vi "Handle Last Ack Core.vi"(4 "error in (no error)":errorcluster, 6 "Last Ack":refnum<class "Last Ack.lvclass">, 7 "TestStand Controller in":refnum<class "Controller API.lvclass">) -> (0 "error out":errorcluster, 3 "TestStand Controller out":refnum<class "Controller API.lvclass">)   [LabVIEW 2016, in "Controller API.lvlib" / "Controller API.lvclass"]
doc: "(<B>Filename</B>: Actor Framework.lvlib:Actor.lvclass:Handle Last Ack Core.vi)\n\nDefines how the caller actor responds to the Last Ack message from a nested actor. The Last Ack message is the final message a nested actor sends to its caller before it shuts down. The message contains information about the final state of the nested actor.\n\nBy default, this method does nothing except return any error the nested actor sent. A descendant class may override this method to define behavior."
uses:
  <userlib>/Measurement Utility API/Controller API.lvclass
  <vilib>/ActorFramework/LastAck/Last Ack.lvclass
  <userlib>/Common Components/Measurement Actor/Measurement.lvclass
  <vilib>/ActorFramework/LastAck/Last Ack.lvclass/Last Ack.ctl
  <userlib>/Common Components/Results/Results.lvclass
  <userlib>/Common Components/Measurement Actor/Measurement.lvclass/Measurement.ctl
  <userlib>/Measurement Utility API/Controller API.lvclass/Controller API.ctl
  <userlib>/Common Components/Controller/Controller.lvclass
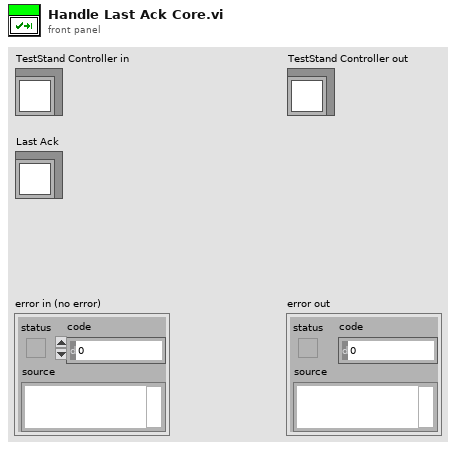
[diagram p1: front panel]
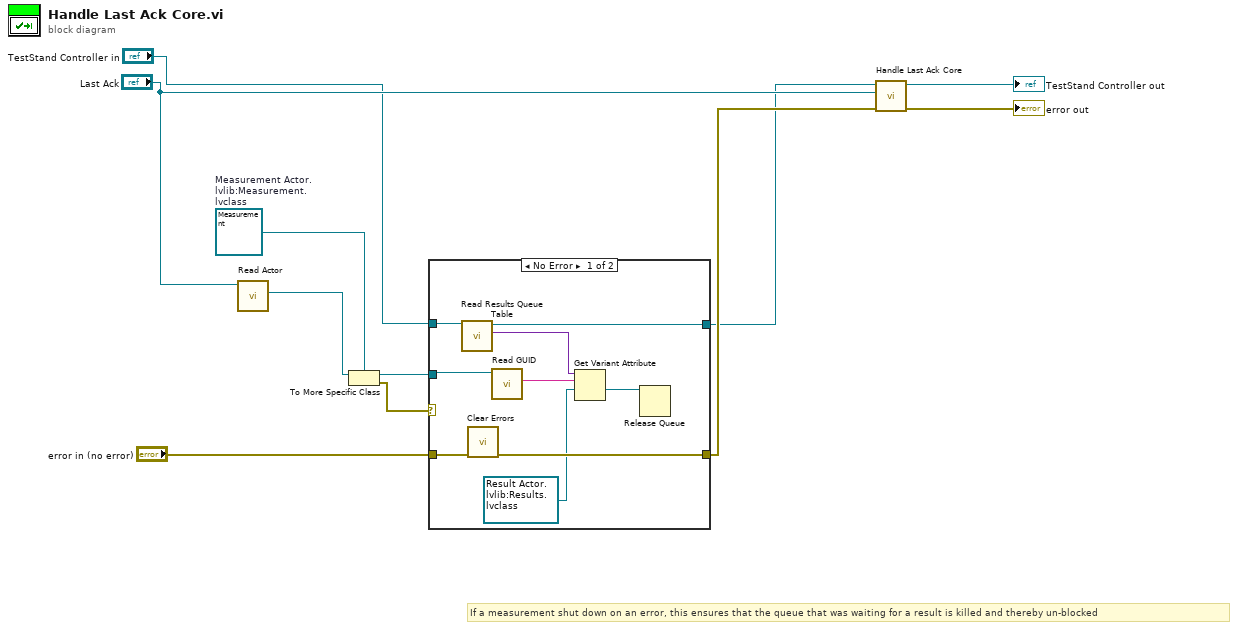
[diagram p0: block diagram]
diagram:
  w7 = refnum<class "Measurement.lvclass"> refnum  # Measurement Actor.lvlib:Measurement.lvclass
  # "If a measurement shut down on an error, this ensures that the queue that was waiting for a result is killed and thereby un-blocked"
  n1 = call <vilib>:"Read Actor.vi"("Last Ack"="Last Ack") -> ("Actor"=w8:refnum<class "Actor.lvclass">)  [unwired: 10 in]
  n2 = To More Specific Class(target class=w7, reference=w8) -> (specific class reference=w5:refnum<class "Measurement.lvclass">, error out=w6:errorcluster)  [unwired: 1 in]
  n3 = case shown="No Error" w6 {
    tunnel: w5 -> [w20 _]
    tunnel: "error in (no error)" -> [w19 w22]
    tunnel: [w18 w22] -> w3
    tunnel: "TestStand Controller in" -> [w17 w21]
    tunnel: [w14 w21] -> w1
    frame No Error {
      n4 = call <userlib>:"Read Results Queue Table.vi"("TestStand Controller in"=w17) -> ("Results Queue Table"=w16:variant, "TestStand Controller out"=w14:refnum<class "Controller API.lvclass">)  [unwired: 8 in, 1 out]
      n5 = call <vilib>:"Clear Errors.vi"("error in (no error)"=w19) -> ("error out"=w18:errorcluster)  [unwired: 5 in, 1 out]
      n6 = call <userlib>:"Read GUID.vi"("Measurement in"=w20) -> ("GUID"=w15:string)  [unwired: 8 in, 2 out]
      n7 = Get Variant Attribute(Variant=w16, name=w15, default value (empty Variant)=refnum<queue> refnum ("Results Queue")) -> (value=w12:refnum<queue>)  [unwired: 1 in, 3 out]
      n8 = Release Queue(queue=w12) -> ()  [unwired: 2 in, 3 out]
    }
    frame Error {
    }
  }
  n9 = call-parent "Handle Last Ack Core.vi"("error in (no error)"=w3, "Last Ack"="Last Ack", "Controller in"=w1) -> ("error out"=→"error out":errorcluster, "Controller out"=→"TestStand Controller out":refnum<class "Controller API.lvclass">)  [unwired: 3 in]
